vi "le_escreve_analogico.vi"() -> ()   [LabVIEW 2020]
uses:
  <vilib>/DAQmx/write.llb/DAQmx Write (Analog DBL 1Chan 1Samp).vi
  <vilib>/DAQmx/read.llb/DAQmx Read (Analog DBL 1Chan 1Samp).vi
  <vilib>/DAQmx/create/channels.llb/DAQmx Create Channel (AO-Voltage-Basic).vi
  <vilib>/DAQmx/create/channels.llb/DAQmx Create Channel (AI-Voltage-Basic).vi
  <vilib>/DAQmx/miscellaneous.llb/DAQmx Fill In Error Info.vi
panel:
  in  "physical channels 2":tag
  out "out":dbl
  out "task out 3":refnum<k21>
  out "task out 2":refnum<k21>
  in  "task in 2":refnum<k21>
  in  "physical channels":tag
  in  "task in":refnum<k21>
  in  "in":dbl(slide) scale=0.0..10.0
  out "error out":errorcluster
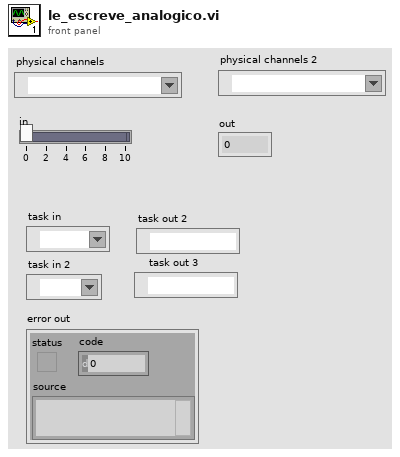
[diagram p1: front panel]
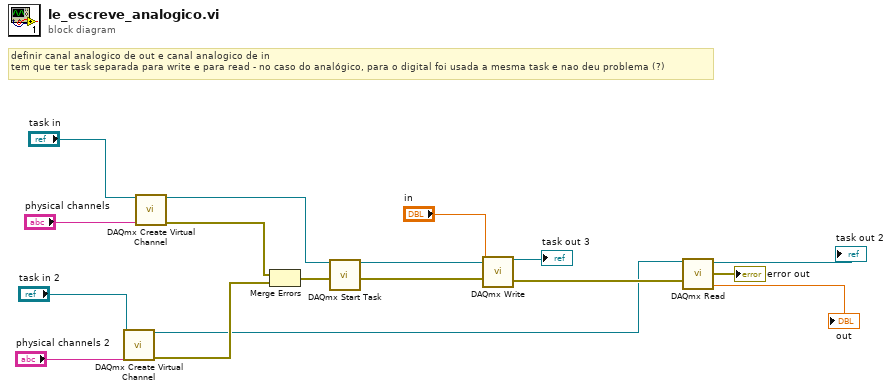
[diagram p0: block diagram]
diagram:
  # "definir canal analogico de out e canal analogico de in\ntem que ter task separada para write e para read - no caso do analógico, para o digital foi usada a mesma task e nao deu problema (?)"
  n1 = call-poly <vilib>:"DAQmx Create Virtual Channel.vi"("task in"="task in 2", "physical channels"="physical channels 2") -> ("task out"=w1:refnum<k21>, "error out"=w8:errorcluster)  [unwired: 12 in]
  n2 = call-poly <vilib>:"DAQmx Create Virtual Channel.vi"("task in"="task in", "physical channels"="physical channels") -> ("task out"=w13:refnum<k21>, "error out"=w17:errorcluster)  [unwired: 12 in]
  n3 = Merge Errors(w17, w8) -> (w16:errorcluster)
  n4 = call <vilib>:"DAQmx Start Task.vi"("task/channels in"=w13, "error in"=w16) -> ("task out"=w12:refnum<k21>, "error out"=w15:errorcluster)  [unwired: 12 in]
  n5 = call-poly <vilib>:"DAQmx Write.vi"("task/channels in"=w12, "data"="in", "error in"=w15) -> ("task out"=→"task out 3":refnum<k21>, "error out"=w4:errorcluster)  [unwired: 10 in, 1 out]
  n6 = call-poly <vilib>:"DAQmx Read.vi"("task/channels in"=w1, "error in"=w4) -> ("task out"=→"task out 2":refnum<k21>, "data"=→"out":dbl, "error out"=→"error out":errorcluster)  [unwired: 11 in]
